vi "ACQ PostProces1.vi"(5 "ACQ full DATA file path":path caption="File path", 7 "Addresses Cluster":T1={"ENA1"=FALSE, "IP address 1"="172.16.14.22", "ENA2"=FALSE, "IP address 2"="172.16.14.23"}, 8 "Chip ID list 2":u16[](array[numeric]) format="%.0x", 9 "Chip ID list 1":u16[](array[numeric]) format="%.0x", 10 "events per file in":u32, 11 "file sufix num. in":u32) -> (0 "summary temp B":u32[][](array[numeric]), 1 "summary temp A":u32[][](array[numeric]), 2 "events per file out":u32, 3 "file sufix num. out":u32)   [LabVIEW 2015, in "VIPM2.lvlib"]
doc: "PostProcess the ACQ temp files to get the summary temps.\nTotalize the global Summary and update it into disk.\nMerge temp files into ACQ binary file."
uses:
  VIPM2.lvlib
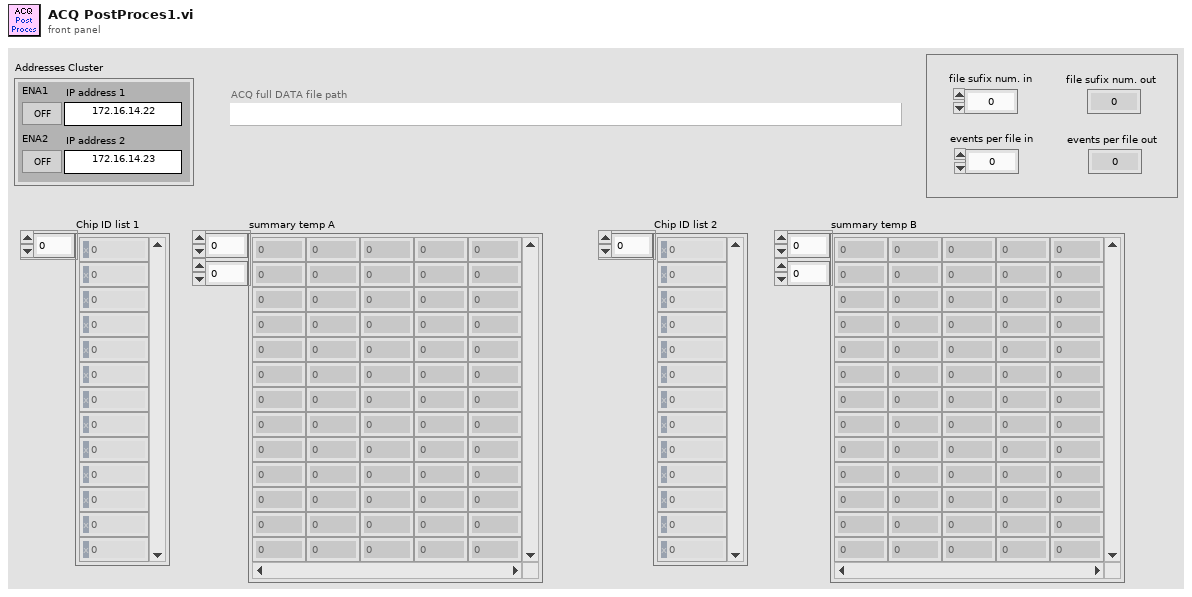
[diagram p1: front panel]
types:
  T1 = cluster{"ENA1":bool, "IP address 1":string, "ENA2":bool, "IP address 2":string}
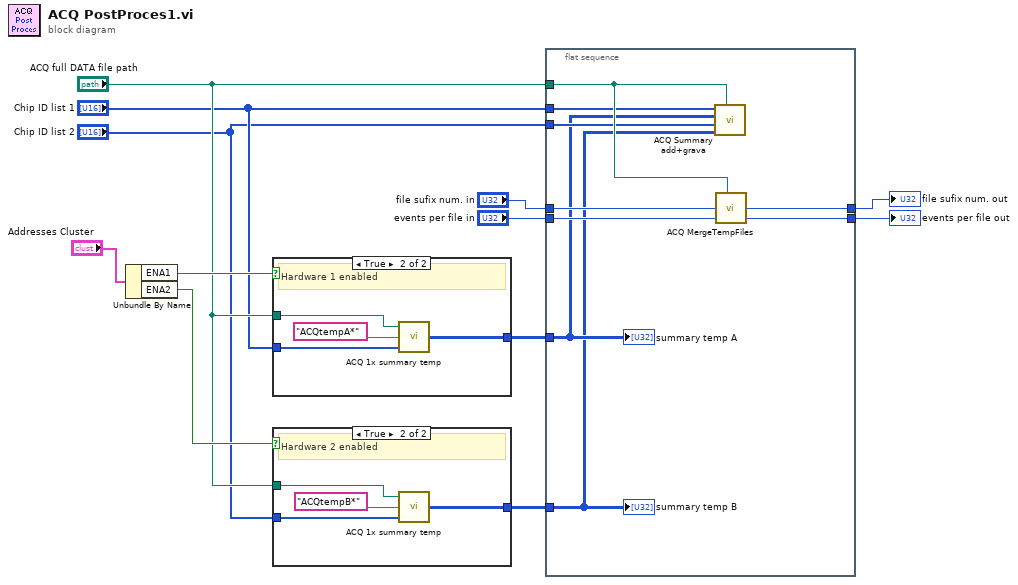
[diagram p0: block diagram]
diagram:
  n1 = Unbundle By Name("Addresses Cluster") -> ("ENA1"=w11:bool, "ENA2"=w10:bool)
  n2 = case shown="True" w11 {
    tunnel: "ACQ full DATA file path" -> [_ w16]
    tunnel: "Chip ID list 1" -> [_ w15]
    tunnel: [_ w13] -> w6
    frame False {
      # "Hardware 1 not enabled"
    }
    frame True {
      # "Hardware 1 enabled"
      n3 = call "ACQ 1x summary temp.vi"("1x ChipID list"=w15, "ACQtemp* pattern"="ACQtempA*", "ACQ full DATA file path"=w16) -> ("1x summary temp out"=w13:u32[][])  [unwired: 2 in]
    }
  }
  n4 = case shown="True" w10 {
    tunnel: "ACQ full DATA file path" -> [_ w20]
    tunnel: "Chip ID list 2" -> [_ w19]
    tunnel: [_ w17] -> w5
    frame False {
      # "Hardware 2 not enabled"
    }
    frame True {
      # "Hardware 2 enabled"
      n5 = call "ACQ 1x summary temp.vi"("1x ChipID list"=w19, "ACQtemp* pattern"="ACQtempB*", "ACQ full DATA file path"=w20) -> ("1x summary temp out"=w17:u32[][])  [unwired: 2 in]
    }
  }
  n6 = flat-sequence {
    tunnel: "ACQ full DATA file path" -> [w29]
    tunnel: "Chip ID list 1" -> [w28]
    tunnel: "Chip ID list 2" -> [w27]
    tunnel: w6 -> [w22]
    tunnel: w5 -> [w21]
    tunnel: "file sufix num. in" -> [w26]
    tunnel: "events per file in" -> [w25]
    tunnel: [w24] -> w2
    tunnel: [w23] -> w1
    frame #0 {
      n7 = call "ACQ Summary add+grava.vi"("ACQ full DATA file path"=w29, "summary temp B"=w21, "ChipID list 2"=w27, "summary temp A"=w22, "ChipID list 1"=w28) -> ()  [unwired: 7 in]
      n8 = call "ACQ MergeTempFiles.vi"("Base file path amb comentaris"=w29, "file sufix num. in"=w26, "Comptador events per file in"=w25) -> ("file sufix num. out"=w23:u32, "Comptador events per file out"=w24:u32)  [unwired: 3 in]
      "summary temp A" <- w22
      "summary temp B" <- w21
    }
  }
  "file sufix num. out" <- w1
  "events per file out" <- w2
